vi "close.vi"(8 "error in":errorcluster, 11 "FPGA Module runtime in":refnum<class "FPGA Module runtime.lvclass">) -> (0 "error out":errorcluster)   [LabVIEW 2017, in "FPGA Module runtime.lvclass"]
doc: "Provides an interface for terminating a module instance. While this interface performs no operations, a child should close and deallocate any open references or memory."
uses:
  FPGA Module runtime.lvclass
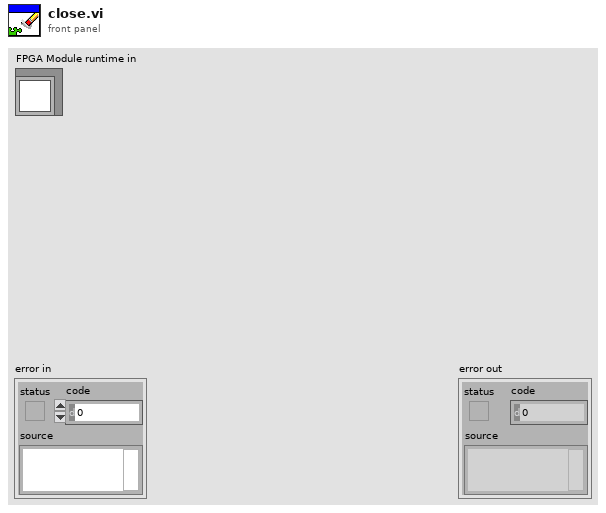
[diagram p1: front panel]
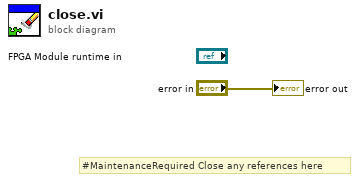
[diagram p0: block diagram]
diagram:
  # "#MaintenanceRequired Close any references here"
  "error out" <- "error in"
